vi "Log Force Sensor Calibration.vi"(8 "error in (no error)":errorcluster, 9 "timed out?":bool, 10 "Force Sensor in":refnum<class "Force Sensor.lvclass">, 11 "array results in":T1) -> (0 "error out":errorcluster, 3 "array results out":T1)   [LabVIEW 2020]
uses:
  Controller Loop/Controller Data.ctl
  Hardware/Sensors/Force Sensors/Force Sensor.lvclass
  Hardware/Sensors/Force Sensors/Force Sensor.lvclass/Force Sensor.ctl
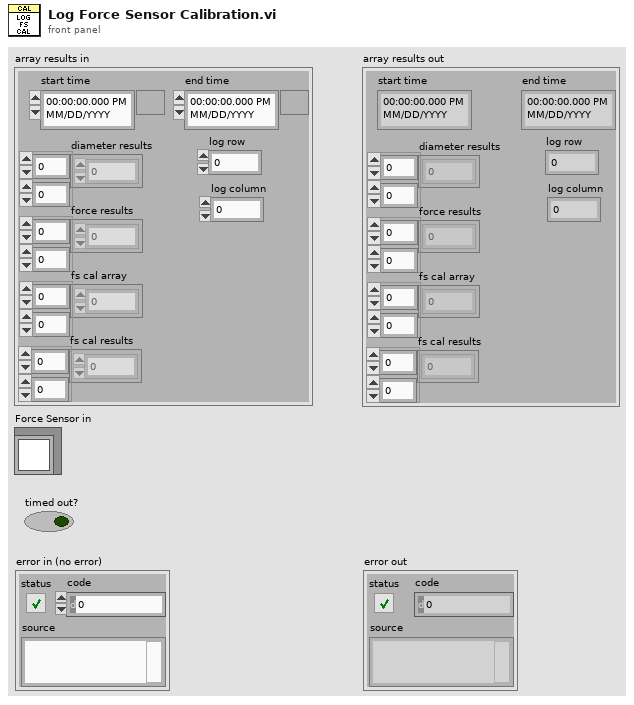
[diagram p1: front panel]
types:
  T1 = typedef "Controller Data.ctl" = cluster{"diameter results":dbl[][], "force results":dbl[][], "fs cal array":dbl[][], "fs cal results":dbl[][], "start time":timestamp, "end time":timestamp, "log row":i32, "log column":i32}
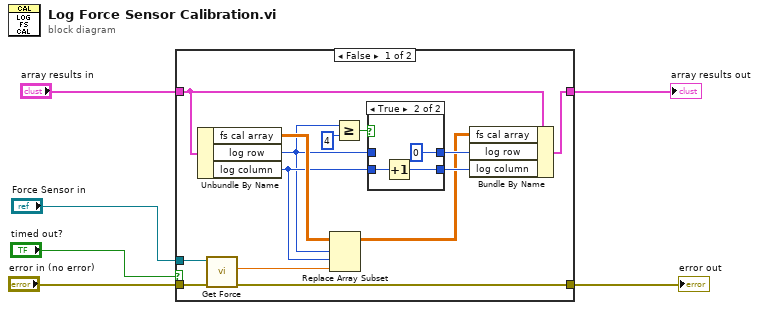
[diagram p0: block diagram]
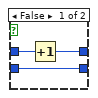
[diagram p2: hidden frame]
diagram:
  n1 = case shown="False" "timed out?" {
    tunnel: "error in (no error)" -> [w20 w28]
    tunnel: [w16 w28] -> w3
    tunnel: "Force Sensor in" -> [w19 _]
    tunnel: "array results in" -> [w18 w27]
    tunnel: [w17 w27] -> w6
    frame False {
      n2 = Unbundle By Name(w18) -> ("fs cal array"=w15:dbl[][], "log row"=w7:i32, "log column"=w12:i32)
      n3 = call "Get Force.vi"("error in (no error)"=w20, "Force Sensor in"=w19) -> ("error out"=w16:errorcluster, "force (V)"=w14:dbl)  [unwired: 7 in, 1 out]
      n4 = Replace Array Subset(array=w15, new element=w14, index (row)=w7, index (col)=w12) -> (w9:dbl[][])
      n5 = Greater Or Equal?(x=w7, y=4 ("x")) -> (x >= y?=w13:bool)
      n6 = case shown="True" w13 {
        tunnel: w7 -> [w23 _]
        tunnel: w12 -> [w21 w26]
        tunnel: [w21 w25] -> w11
        tunnel: [w22 0 ("x+1")] -> w10
        frame False {
          n7 = Increment(x=w23) -> (x+1=w22:i32)
        }
        frame True {
          n8 = Increment(x=w26) -> (x+1=w25:i32)
        }
      }
      n9 = Bundle By Name(cluster=w18, "fs cal array"=w9, "log row"=w10, "log column"=w11) -> (w17:T1)
    }
    frame True {
      # "Do nothing if timed out"
    }
  }
  "array results out" <- w6
  "error out" <- w3
